vi "test1.vi"() -> ()   [LabVIEW 2016]
panel:
  out "MAIN STOP 3":bool
  in  "MAIN STOP 2":bool
  in  "MAIN STOP":bool
  out "x+1 2":i32
  out "x+1":i32
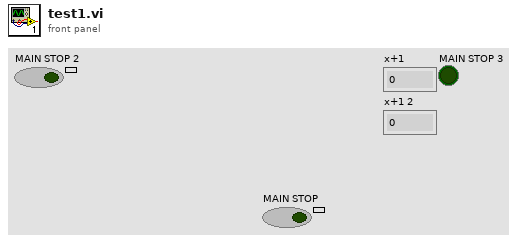
[diagram p1: front panel]
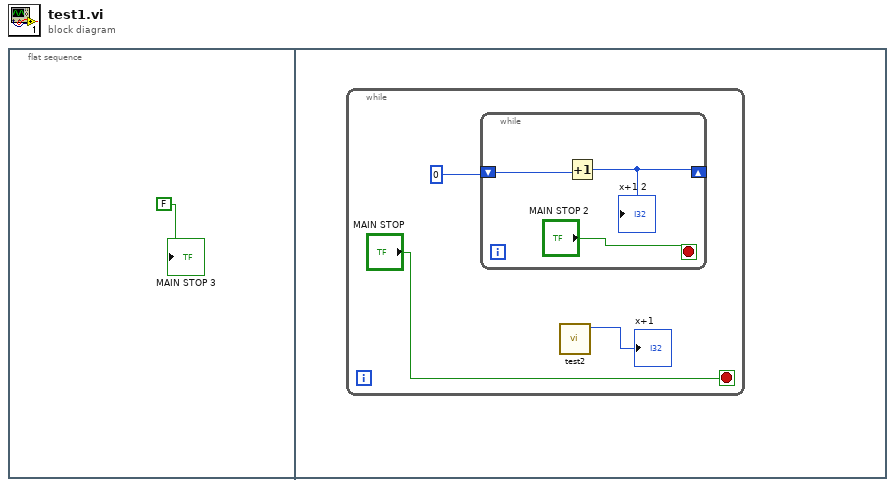
[diagram p0: block diagram]
diagram:
  n1 = flat-sequence {
    frame #0 {
      "MAIN STOP 3" <- FALSE ("MAIN STOP")
    }
    frame #1 {
      n2 = while {
        stop <- "MAIN STOP" stop-if-true
        n3 = while {
          shift-right: [w6] -> _
          shift-left: 0 -> [w7]
          stop <- "MAIN STOP 2" stop-if-true
          n4 = Increment(x=w7) -> (x+1=w6:i32)
          "x+1 2" <- w6
        }
        n5 = call "test2.vi"() -> ("x+1"=→"x+1":i32)  [unwired: 11 in]
      }
    }
  }
